vi "InitCluster.vi"(8 "ErrorArray in":errorcluster[](array[cluster]), 10 "ClusterRefArray":refnum<vi>[](array[refnum]), 11 "IniFileRef in":T1) -> (0 "ErrorArray Out":errorcluster[](array[cluster]), 3 "IniFileRef out":T1)   [LabVIEW 2014, in "Ini_lib.lvlib"]
uses:
  Ini_lib.lvlib
  <vilib>/Utility/config.llb/Config Data RefNum.ctl
  <userlib>/NIST/NISTErrorLib/NISTErrorLib.lvlib
  <vilib>/Utility/config.llb/NI_LVConfig.lvlib
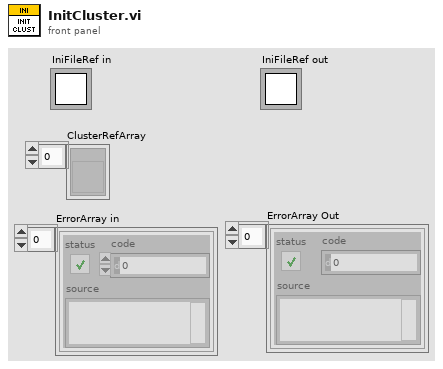
[diagram p1: front panel]
types:
  T1 = typedef "NI_LVConfig.lvlib/Config Data RefNum.ctl" = refnum<k1>
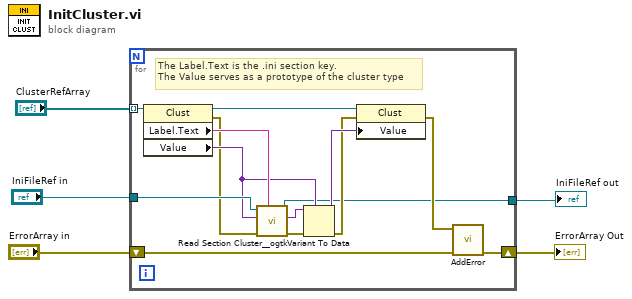
[diagram p0: block diagram]
diagram:
  n1 = for {
    tunnel: "ClusterRefArray" -> [w18] mode=indexing
    tunnel: "IniFileRef in" -> [w19]
    shift-right: [w7] -> w2
    shift-left: "ErrorArray in" -> [w8]
    tunnel: [w6] -> w1
    # "The Label.Text is the .ini section key.\nThe Value serves as a prototype of the cluster type"
    n2 = property class="Clust"(reference=w18) -> (reference out=w13:refnum<vi>, error out=w11:errorcluster, "Label.Text"=w17:string, "Value"=w14:variant)  [unwired: 1 in]
    n3 = call <userlib>:"Read Section Cluster__ogtk.vi"("section (optional)"=w17, "error in (no error)"=w11, "Section Formatted Cluster Type"=w14, "refnum"=w19) -> ("error out"=w16:errorcluster, "Section Formatted Cluster"=w15:variant, "dup refnum"=w6:T1)  [unwired: 3 in, 2 out]
    n4 = Variant To Data(error in=w16, type=w14, Variant=w15) -> (data=w12:variant, error out=w10:errorcluster)
    n5 = property class="Clust"(reference=w13, error in=w10, "Value"=w12) -> (error out=w9:errorcluster)  [unwired: 1 out]
    n6 = call <userlib>:"AddError.vi"("ErrorArray"=w8, "error in (no error)"=w9) -> ("ErrorArray"=w7:errorcluster[])  [unwired: 8 in, 1 out]
  }
  "ErrorArray Out" <- w2
  "IniFileRef out" <- w1
